vi "LoadController.vi"(8 "error in (no error)":errorcluster, 10 "Actor In":refnum<class "Actor.lvclass">, 11 "DemoDAQ in":refnum<class "DemoDAQ.lvclass">) -> (0 "error out":errorcluster, 3 "DemoDAQ out":refnum<class "DemoDAQ.lvclass">)   [LabVIEW 2020, in "DemoDAQ.lvlib" / "DemoDAQ.lvclass"]
uses:
  DemoDAQ.lvclass
  ViewController/QPDController/QPDController.lvclass
  Hardware Abstraction Layer/Component/DAQ/DAQ/DAQ.lvclass
  C:/Program Files/National Instruments/LabVIEW 2020/vi.lib/ActorFramework/Actor/Actor.lvclass
  <vilib>/ActorFramework/Actor/Actor.lvclass
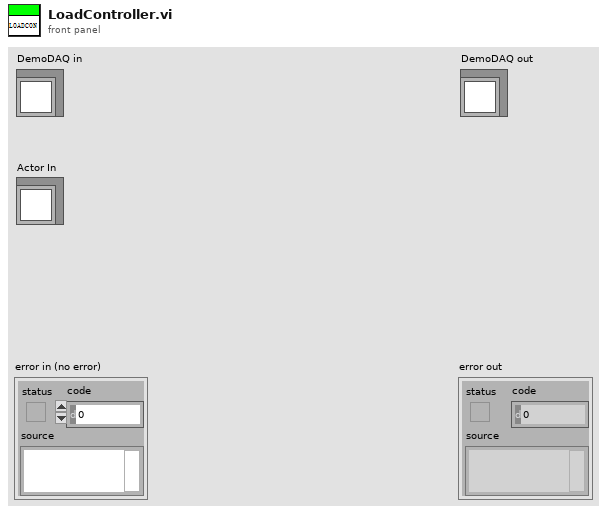
[diagram p1: front panel]
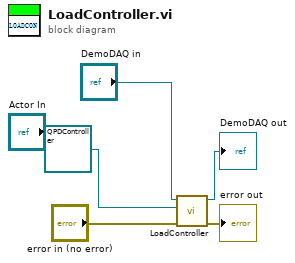
[diagram p0: block diagram]
diagram:
  n1 = call-parent "LoadController.vi"("error in (no error)"="error in (no error)", "Actor In"=refnum<class "QPDController.lvclass"> refnum ("QPDController.lvlib:QPDController.lvclass"), "Device in"="DemoDAQ in") -> ("error out"=→"error out":errorcluster, "Device out"=→"DemoDAQ out":refnum<class "DemoDAQ.lvclass">)  [unwired: 7 in]
